vi "MM6.InitScanDevs.vi"(0 "i ref in":refnum<vi>, 2 "InitObjs":string[](array[string]), 3 "ms timeout (10000)":i32=10000, 5 "error in (no error)":errorcluster) -> (14 "i ref out":refnum<vi>, 16 "InitObjs out":string[](array[string]), 17 "timed out":bool, 19 "error out":errorcluster)   [LabVIEW 2014, in "MM6.lvlib"]
doc: "Initializes the scan devices."
uses:
  MM6.lvlib
  LEBITLib/LEBITLib.lvlib
  CS_Core/BaseProcess/BaseProcess.lvlib
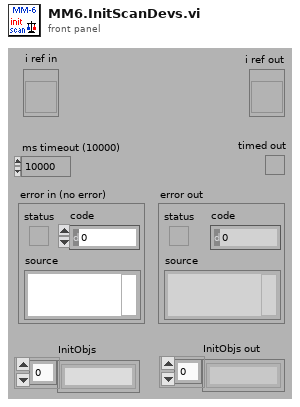
[diagram p1: front panel]
types:
  T1 = typedef "MM6.lvlib/MM6.i attribute.ctl" = cluster{"ConfigData":T2, "UsedObjs":string[], "ActScanStep":i32[], "AbortRequest":bool, "StopRequest":bool, "# cycles":i32, "Connected":bool, "MMStatus":T17, "# data":i32, "DIMServices":cluster{"MM6StatusString":string, "MM6StatusID":i32, "discArchiver":string, "discArchiverID":i32, "eventBuilder":string, "eventBuilderID":i32, "GUIIDString":string, "GUIIDStringID":i32}, "dataFile":string, "ExtraDataSets":T18, "PGRunning":T19}
  T2 = typedef "LEBITDefs.lvlib/LEBITDefs.ConfigData.ctl" = cluster{"GenConfig":T3, "Configs":T5[]}
  T3 = typedef "LEBITDefs.lvlib/LEBITDefs.GenConfig.ctl" = cluster{"Mode":i32, "Logs":T4[]}
  T4 = typedef "LEBITDefs.lvlib/LEBITDefs.Log.ctl" = cluster{"Name":string, "FctName":string, "Special":string}
  T5 = typedef "LEBITDefs.lvlib/LEBITDefs.OneConfig.ctl" = cluster{"MCA":T6, "Timing":T7, "Scans":T10[], "FreqDevs":T11[], "CleanDev":T12, "NrCycles":i32, "Specials":T14[], "Delays":T15[], "DAC":T16}
  T6 = typedef "LEBITDefs.lvlib/LEBITDefs.MCA.ctl" = cluster{"Name":string, "Address":string, "NrChannels":i32, "Gate":i32, "NrPipse":i32}
  T7 = typedef "LEBITDefs.lvlib/LEBITDefs.Timing.ctl" = cluster{"TimeTables":cluster{"TimeTable":T8}[], "Memories":T9[], "ScanX":string, "ScanY":string}
  T8 = typedef "LEBITDefs.lvlib/LEBITDefs.Timetable.ctl" = dbl[]
  T9 = typedef "LEBITDefs.lvlib/LEBITDefs.Memory.ctl" = cluster{"Device":string, "ExtTrig":bool, "TT2Use":i32, "PatternTable":string[]}
  T10 = typedef "LEBITDefs.lvlib/LEBITDefs.ScanDev.ctl" = cluster{"Name":string, "FctName":string, "Values":dbl[], "NrScanVals":i32, "Special":string}
  T11 = typedef "LEBITDefs.lvlib/LEBITDefs.FreqDev.ctl" = cluster{"Name":string, "Amp":dbl, "CenterFreq":dbl, "Time":dbl}
  T12 = typedef "LEBITDefs.lvlib/LEBITDefs.CleanDev.ctl" = cluster{"Name":string, "CleanData":T13[]}
  T13 = typedef "LEBITDefs.lvlib/LEBITDefs.CleanDataType.ctl" = cluster{"Amp":dbl, "Center":dbl, "Plus":dbl, "Minus":dbl, "Time":dbl}
  T14 = typedef "LEBITDefs.lvlib/LEBITDefs.Special.ctl" = cluster{"Name":string, "FctName":string, "VerySpecial":string, "Data":dbl}
  T15 = typedef "LEBITDefs.lvlib/LEBITDefs.Delay.ctl" = cluster{"Name":string, "Delay":dbl}
  T16 = typedef "LEBITDefs.lvlib/LEBITDefs.DAC.ctl" = cluster{"Name":string, "Step1":i32, "Step2":i32}
  T17 = typedef "MM6.lvlib/MM6.status.ctl" = enum16{"loaded", "load_error", "config", "config_error", "init", "init_error", "data_reset", "data_reset_error", "running", "start_error", "run_error", "abort_requested", "aborted", "stop_requested", "stopped", "stop_error", "Connected", "NOTConnected"}
  T18 = typedef "LEBITDefs.lvlib/LEBITDefs.ExtraData.ctl" = cluster{"Ions":cluster{"ExcitIonMass":string, "ExcitIonCharge":i32, "CleanIons":cluster{"CleanIonMass":string, "CleanIonCharge":i32}[]}, "TimingDescription":cluster{"TimeTableDescription":cluster{"Times":string[]}[], "PatternTableDescription":cluster{"Pattern":string[]}[]}, "ScanUnits":string[]}[]
  T19 = typedef "PPG_ABC.lvlib/PPG_ABC.PG_Running.ctl" = i32
  T20 = typedef "CoreDefs.rawDataType.ctl" = i8[]
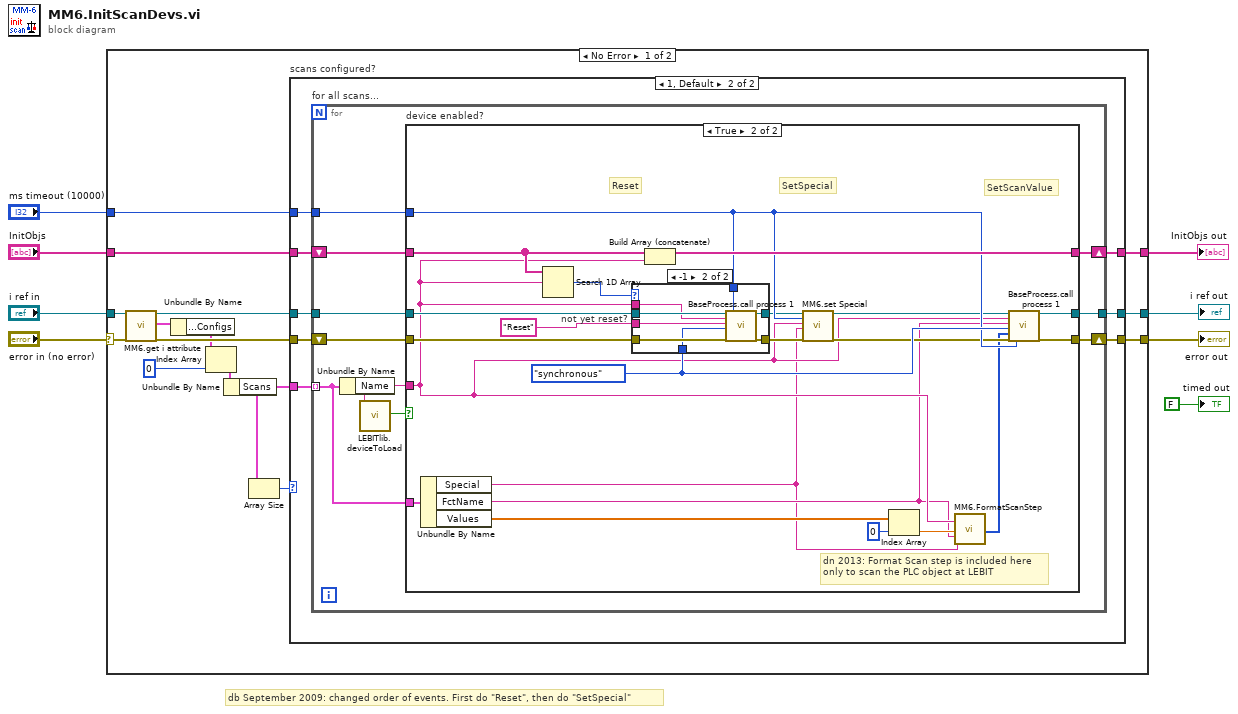
[diagram p0: block diagram]
diagram:
  # "db September 2009: changed order of events. First do \"Reset\", then do \"SetSpecial\""
  n1 = case shown="No Error" "error in (no error)" {
    selector: "error in (no error)" -> [w16 w80]
    tunnel: "i ref in" -> [w21 w81]
    tunnel: [w18 w81] -> w7
    tunnel: [w17 w80] -> w6
    tunnel: "InitObjs" -> [w15 w82]
    tunnel: [w14 w82] -> w2
    tunnel: "ms timeout (10000)" -> [w9 _]
    frame No Error {
      n2 = call "MM6.get i attribute.vi"("i ref in"=w21, "error in (no error)"=w16) -> ("i ref out"=w20:refnum<vi>, "i attribute"=w13:T1, "error out"=w19:errorcluster)  [unwired: 15 in]
      n3 = Unbundle By Name(w13) -> ("ConfigData.Configs"=w12:T5[])
      n4 = Index Array(array=w12, index=0) -> (element=w11:T5)
      n5 = Unbundle By Name(w11) -> ("Scans"=w22:T10[])
      n6 = Array Size(array=w22) -> (size(s)=w23:i32)
      n7 = case "scans configured?" shown="1, Default" w23 {
        tunnel: w22 -> [_ w34]
        tunnel: w20 -> [w26 w33]
        tunnel: [w26 w32] -> w18
        tunnel: w19 -> [w25 w31]
        tunnel: [w25 w30] -> w17
        tunnel: w15 -> [w24 w29]
        tunnel: [w24 w28] -> w14
        tunnel: w9 -> [_ w27]
        frame 0 {
        }
        frame 1, Default {
          n8 = for "for all scans..." {
            tunnel: w34 -> [w42] mode=indexing
            tunnel: w33 -> [w44]
            tunnel: [w43] -> w32
            shift-right: [w40] -> w30
            shift-left: w31 -> [w41]
            shift-right: [w38] -> w28
            shift-left: w29 -> [w39]
            tunnel: w27 -> [w35]
            n9 = Unbundle By Name(w42) -> ("Name"=w37:string)
            n10 = call "LEBITlib.deviceToLoad.vi"("DeviceName"=w37) -> ("DeviceIsToLoad"=w36:bool)
            n11 = case "device enabled?" shown="True" w36 {
              tunnel: w44 -> [w47 w58]
              tunnel: [w47 w68] -> w43
              tunnel: w41 -> [w46 w57]
              tunnel: w37 -> [_ w50]
              tunnel: [w46 w65] -> w40
              tunnel: w42 -> [_ w69]
              tunnel: w39 -> [w45 w67]
              tunnel: [w45 w66] -> w38
              tunnel: w35 -> [_ w59]
              frame False {
              }
              frame True {
                w60 = enum16{"simple", "synchronous", "asynchronous"}."synchronous" ("CallType")
                # "dn 2013: Format Scan step is included here\nonly to scan the PLC object at LEBIT"
                # "SetScanValue"
                # "Reset"
                # "SetSpecial"
                n12 = Unbundle By Name(w69) -> ("Special"=w48:string, "FctName"=w49:string, "Values"=w63:dbl[])
                n13 = Search 1D Array(1D array=w67, element=w50) -> (index of element=w64:i32)  [unwired: 1 in]
                n14 = case "not yet reset?" shown="-1" w64 {
                  tunnel: w58 -> [w71 w79]
                  tunnel: w57 -> [w70 w78]
                  tunnel: [w71 w77] -> w56
                  tunnel: [w70 w76] -> w53
                  tunnel: w59 -> [_ w75]
                  tunnel: w50 -> [_ w74]
                  tunnel: "Reset" ("Selector") -> [_ w73]
                  tunnel: w60 -> [_ w72]
                  frame 0, Default {
                  }
                  frame -1 {
                    n15 = call "BaseProcess.call process 1.vi"("i ref in"=w79, "Object"=w74, "Selector"=w73, "CallType"=w72, "error in (no error)"=w78, "timeout (ms)"=w75) -> ("i ref out"=w77:refnum<vi>, "error out"=w76:errorcluster)  [unwired: 11 in, 1 out]
                  }
                }
                n16 = Build Array (concatenate)(w67, w50) -> (w66:string[])
                n17 = call "MM6.set Special.vi"("i ref in"=w56, "ms timeout (10000)"=w59, "Object"=w50, "Special"=w48, "error in (no error)"=w53) -> ("i ref out"=w55:refnum<vi>, "error out"=w54:errorcluster)  [unwired: 12 in, 1 out]
                n18 = Index Array(array=w63, index=0) -> (element=w51:dbl)
                n19 = call "MM6.FormatScanStep.vi"("Name"=w50, "Value"=w51, "FctName"=w49, "SetSpecial"=w48) -> ("byteArray out"=w52:T20)  [unwired: 14 in, 1 out]
                n20 = call "BaseProcess.call process 1.vi"("i ref in"=w55, "Object"=w50, "Selector"=w49, "CallType"=w60, "Data"=w52, "error in (no error)"=w54, "timeout (ms)"=w59) -> ("i ref out"=w68:refnum<vi>, "error out"=w65:errorcluster)  [unwired: 10 in, 1 out]
              }
            }
          }
        }
      }
    }
    frame Error {
    }
  }
  "error out" <- w6
  "i ref out" <- w7
  "InitObjs out" <- w2
  "timed out" <- FALSE ("timed out")
